vi "Vision Processing.vi"(4 "error in (no error)":errorcluster, 7 "Image Size":T1=enum."320x240") -> ()   [LabVIEW 2015]
doc: "This VI runs in parallel to other tasks. It gets images from the camera, processes them for color or shape and use that information to affect robot behavior."
uses:
  Support Vision Code/Camera Types.ctl
  <vilib>/Rock Robotics/WPI/Camera/WPI_CameraImageSize.ctl
  <userlib>/836-Library/System/QCP Support Code/QCP_Get_DBL.vi
  <userlib>/836-Library/System/QCP Support Code/QCP_Get_STR.vi
  <vilib>/Rock Robotics/Network Tables/NT Read Boolean.vi
  <userlib>/836-Library/System/QCP Support Code/QCP_Set_DBL.vi
  <vilib>/Rock Robotics/Network Tables/NT Write String.vi
  <vilib>/Rock Robotics/Network Tables/NT Write Number.vi
  <vilib>/Rock Robotics/Network Tables/NT Read Number.vi
  <vilib>/Rock Robotics/Network Tables/NT Read String.vi
  <vilib>/Rock Robotics/Network Tables/NT Write Boolean.vi
  Robot Global Data.vi
  <vilib>/vision/NI_Vision_Development_Module.lvlib
panel:
  out "Right Target":dbl
  out "Left Target":dbl
  out "Target Angle":dbl
  in  "Sideways Camera":bool
  in  "Boresight":dbl format="%#_13g"
  out "Found Targets":T2(array[cluster])=[{"Bounding box"={"left"=112.0, "top"=150.0, "right"=139.0, "bottom"=174.0}, "Aspect Ratio"=70.3125, "Area to CH"=96.83972911963883, "X Mask"=77.77777777777779, "Y Mask"=70.83333333333334, "Moment"=69.2156660279794}]
  out "FPS":dbl=5.212996497577636
  out "Qualified Particles":i32=2
  in  "Score Threshold":dbl=70.0
  in  "Aspect Fudge Factor":dbl=1.0
  in  "Min Score Threshold":dbl=75.0
  in  "Camera Type":T3=enum."MS HD3000 square"
  in  "Emphasize Limit Tests":bool
  out "Masked":T4(plugin-control)
  out "Original Image":T4(plugin-control)
  in  "Display Original":bool=TRUE
  out "Sorted Particle Scores":T5(array[cluster])=[{"Rectangle px"={"Numeric"=112.0, "Numeric 2"=150.0, "Numeric 3"=139.0, "Numeric 5"=174.0}, "Aspect Ratio"=70.3125, "Area to CH"=96.83972911963883, "X"=77.77777777777779, "Y"=70.83333333333334, "Moment Factor"=69.2156660279794}] {"Moment Factor" format="%#_3g"; "Aspect Ratio" format="%#_3g"; "Area to CH" format="%#_3g"; "X" format="%#_3g"; "Y" format="%#_3g"}
  out "Detected Targets":T6(array[cluster])=[{"Distance (ft)"=26.324888830153935, "Center"={-0.3966346153846153, -0.35}, "Normalized Rect"={"Numeric"=-0.46153846153846145, "Numeric 2"=-0.25, "Numeric 3"=-0.33173076923076916, "Numeric 5"=-0.44999999999999996}}] {"Normalized Rect"."Numeric 5" format="%#_2g"; "Normalized Rect"."Numeric 3" format="%#_2g"; "Normalized Rect"."Numeric 2" format="%#_2g"; "Normalized Rect"."Numeric" format="%#_2g"}
  in  "LED Color":T7={"Hue"={152.2312396148097, 250.0}, "Sat"={154.82142857142858, 255.0}, "Val"={100.17857142857143, 255.0}} {"Hue" scale=0.0..255.0 scale format="%#_3g"}
  # "Density Profile"
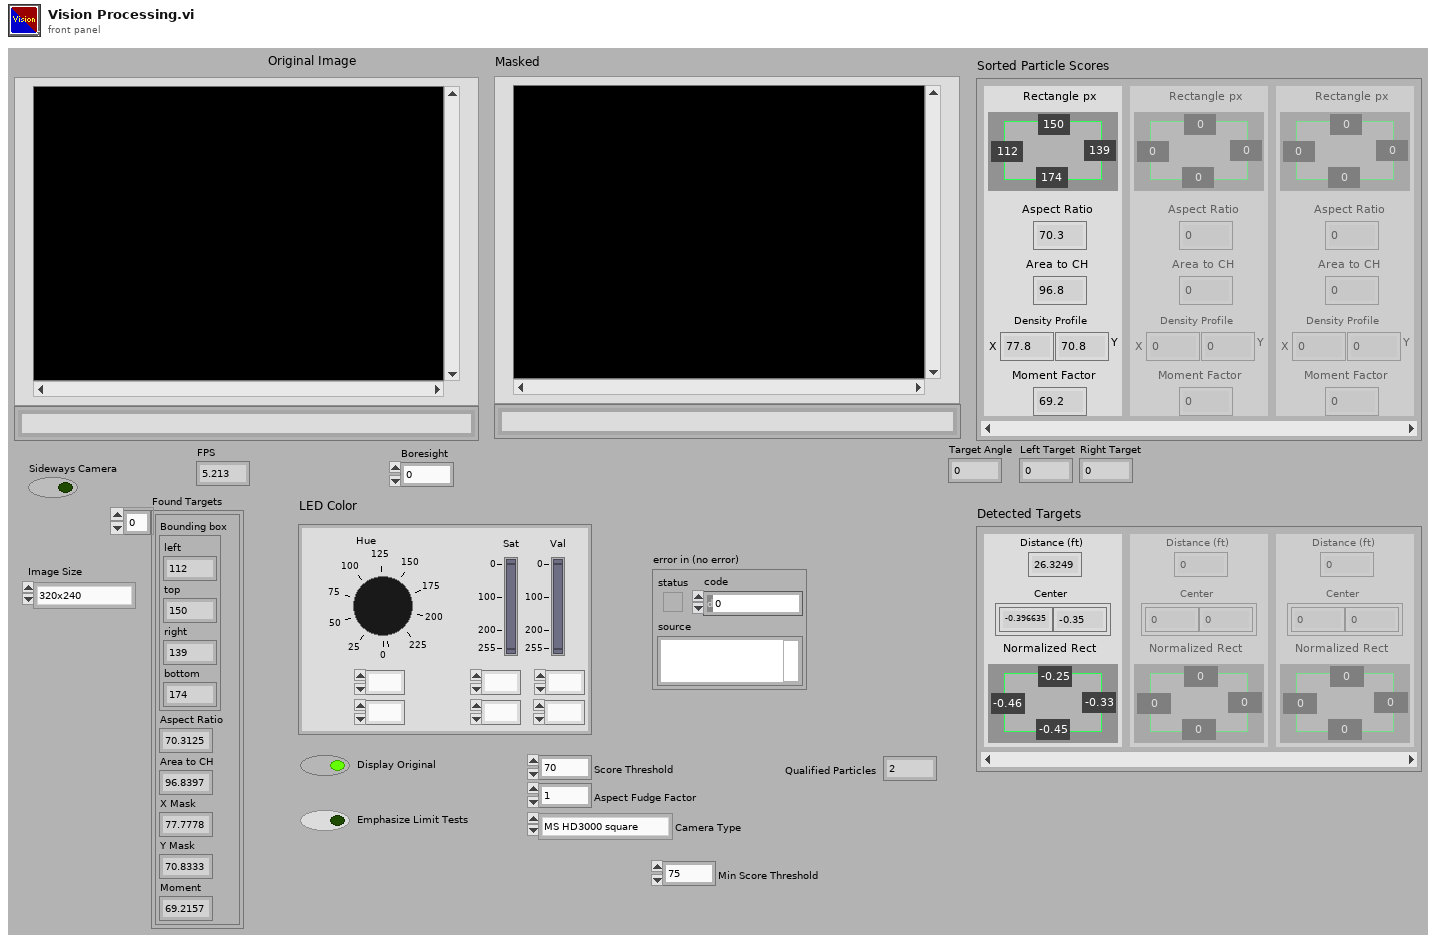
[diagram p1: front panel]
types:
  T1 = typedef "WPI_CameraImageSize.ctl" = enum16{"640x480", "320x240", "160x120", "Custom"}
  T2 = cluster{"Bounding box":cluster{"left":dbl, "top":dbl, "right":dbl, "bottom":dbl}, "Aspect Ratio":dbl, "Area to CH":dbl, "X Mask":dbl, "Y Mask":dbl, "Moment":dbl}[]
  T3 = typedef "Camera Types.ctl" = enum16{"206", "1011", "1013", "MS HD3000 square", "MS HD3000 640x480"}
  T4 = typedef "IMAQ Image.ctl" = refnum<image>
  T5 = cluster{"Rectangle px":cluster{"Numeric":dbl, "Numeric 2":dbl, "Numeric 3":dbl, "Numeric 5":dbl}, "Aspect Ratio":dbl, "Area to CH":dbl, "X":dbl, "Y":dbl, "Moment Factor":dbl}[]
  T6 = cluster{"Distance (ft)":dbl, "Center":cluster{dbl, dbl}, "Normalized Rect":cluster{"Numeric":dbl, "Numeric 2":dbl, "Numeric 3":dbl, "Numeric 5":dbl}}[]
  T7 = cluster{"Hue":cluster{dbl, dbl}, "Sat":cluster{dbl, dbl}, "Val":cluster{dbl, dbl}}
  T8 = typedef "Particle Parameters" = i32
  T9 = typedef "Image Type" = u32
  T10 = typedef "QCP Data Block.ctl" = refnum<data-value>
  T11 = typedef "WPI_CameraDevRef.ctl" = cluster{"Camera Address":string, "CameraStatus":errorcluster}
  T12 = typedef "TDMS Channel Info.ctl" = cluster{"TDMS Data":T13, "TDMS RT FIFO":refnum<k33>}
  T13 = typedef "TDMS RT FIFO Packet.ctl" = cluster{"Group/CMD":i32, "Data":dbl, "Channel":i32}
  T14 = cluster{cluster{"Value Out":dbl, "Value Out":dbl}, cluster{"Value Out":dbl, "Value Out":dbl}, cluster{"Value Out":dbl, "Value Out":dbl}}
  T15 = typedef "Drive Code Bundle.ctl" = cluster{"Sensor Data":T16, "Drive Command rt fifo":refnum<k33>}
  T16 = typedef "Sensor Cluster.ctl" = cluster{"Gyro Data":cluster{"Gyro RT FIFO":refnum<k33>, "Gyro Current":dbl, "Gyro Hold":dbl}, "Encoder Data":cluster{"Encoder RT FIFO":refnum<k33>, "Encoder Current":dbl, "Encoder Hold":dbl}, "Camera Data":cluster{"Camera RT FIFO":refnum<k33>, "Camera Current":T17}}
  T17 = typedef "Camera Cluster.ctl" = cluster{" Angle":dbl, "Valid":bool}
  T18 = cluster{"Rectangle":cluster{"Numeric":dbl, "Numeric 2":dbl, "Numeric 3":dbl, "Numeric 5":dbl}, "L":dbl, "Area to CH":dbl, "X":dbl, "Y":dbl, "Moment Factor":dbl}[]
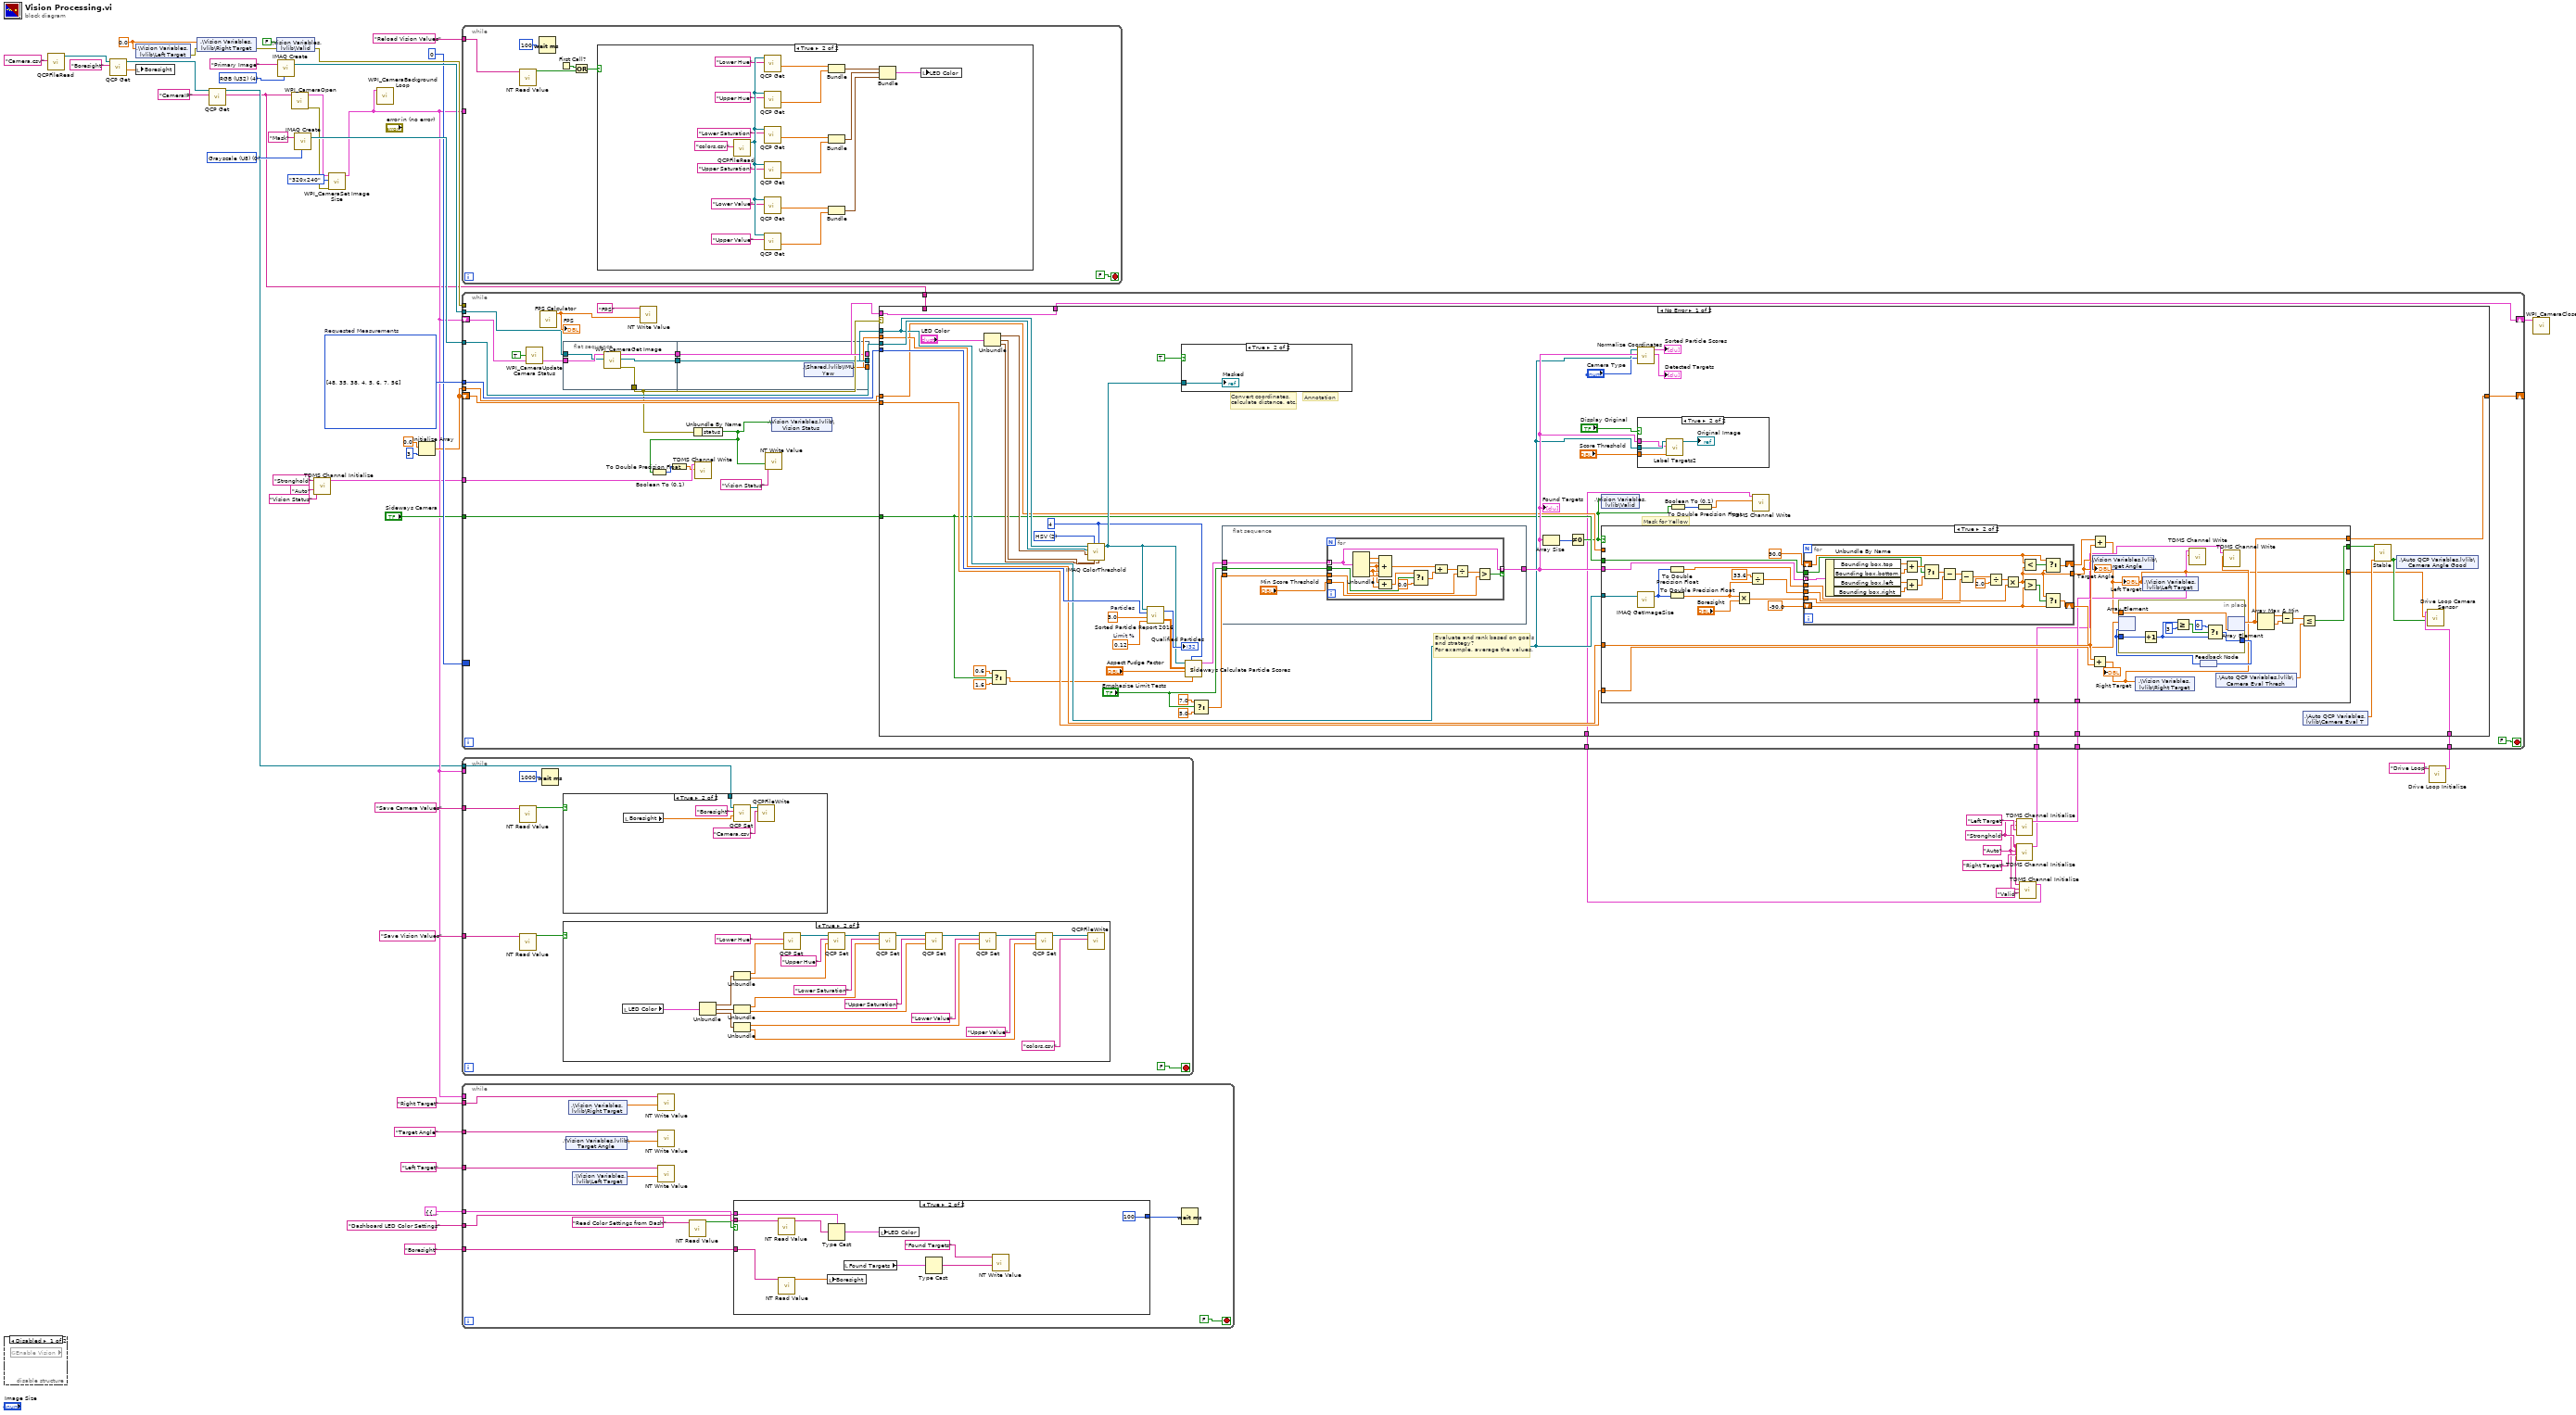
[diagram p0: block diagram]
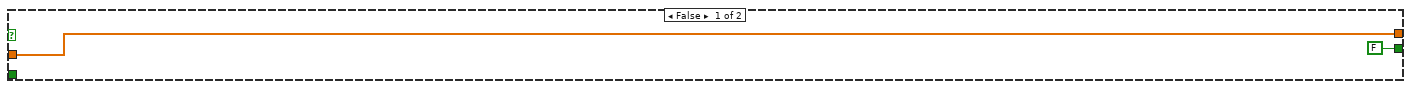
[diagram p5: hidden frame]
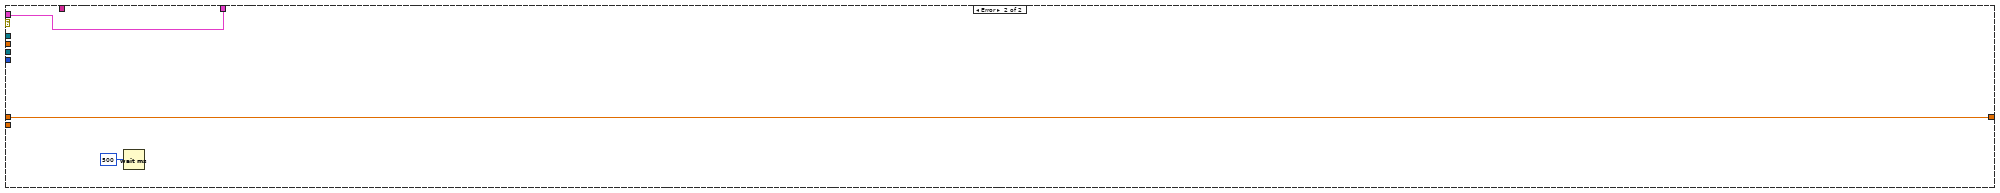
[diagram p6: hidden frame]
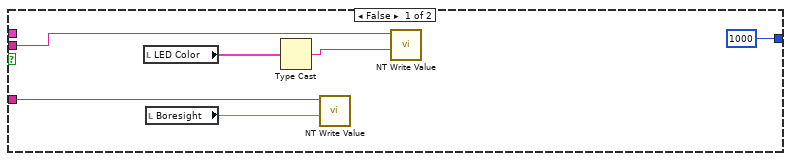
[diagram p7: hidden frame]
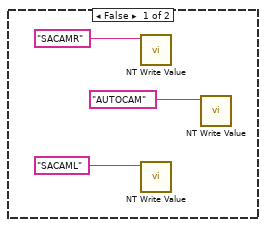
[diagram p8: hidden frame]
diagram:
  w7 = "Auto" ("Group")
  w8 = "Stronghold" ("TDMS Name")
  w30 = T8[] [48, 35, 38, 4, 5, 6, 7, 56] items=["Center of Mass X", "Center of Mass Y", "First Pixel X", "First Pixel Y", "Bounding Rect Left", "Bounding Rect Top", "Bounding Rect Right", "Bounding Rect Bottom", "Max Feret Diameter Start X", "Max Feret Diameter Start Y", "Max Feret Diameter End X", "Max Feret Diameter End Y", "Max Horiz. Segment Length Left", "Max Horiz. Segment Length Right", "Max Horiz. Segment Length Row", "-", "Bounding Rect Width", "Bounding Rect Height", "Bounding Rect Diagonal", "Perimeter", "Convex Hull Perimeter", "Holes' Perimeter", "Max Feret Diameter", "Equivalent Ellipse Major Axis", "Equivalent Ellipse Minor Axis", "Equivalent Ellipse Minor Axis (Feret)", "Equivalent Rect Long Side", "Equivalent Rect Short Side", "Equivalent Rect Diagonal", "Equivalent Rect Short Side (Feret)", "Average Horiz. Segment Length", "Average Vert. Segment Length", "Hydraulic Radius", "Waddel Disk Diameter", "-", "Area", "Holes' Area", "Particle & Holes' Area", "Convex Hull Area", "Image Area", "-", "Number of Holes", "Number of Horiz. Segments", "Number of Vert. Segments", "-", "Orientation", "Max Feret Diameter Orientation", "-", "% Area/Image Area", "% Area/(Particle & Holes' Area)", "Ratio of Equivalent Ellipse Axes", "Ratio of Equivalent Rect Sides", "-", "Elongation Factor", "Compactness Factor", "Heywood Circularity Factor", "Type Factor", "-", "Sum X", "Sum Y", "Sum XX", "Sum XY", "Sum YY", "Sum XXX", "Sum XXY", "Sum XYY", "Sum YYY", "-", "Moment of Inertia XX", "Moment of Inertia XY", "Moment of Inertia YY", "Moment of Inertia XXX", "Moment of Inertia XXY", "Moment of Inertia XYY", "Moment of Inertia YYY", "Norm. Moment of Inertia XX", "Norm. Moment of Inertia XY", "Norm. Moment of Inertia YY", "Norm. Moment of Inertia XXX", "Norm. Moment of Inertia XXY", "Norm. Moment of Inertia XYY", "Norm. Moment of Inertia YYY", "Hu Moment 1", "Hu Moment 2", "Hu Moment 3", "Hu Moment 4", "Hu Moment 5", "Hu Moment 6", "Hu Moment 7"]  # Requested Measurements
  w41 = 0.0 ("Left Target")
  w49 = T9 0 items=["Grayscale (U8)", "Grayscale (I16)", "Grayscale (SGL)", "Complex (CSG)", "RGB (U32)", "HSL (U32)", "RGB (U64)", "Grayscale (U16)"] ("Image Type")
  w52 = T9 4 items=["Grayscale (U8)", "Grayscale (I16)", "Grayscale (SGL)", "Complex (CSG)", "RGB (U32)", "HSL (U32)", "RGB (U64)"] ("Image Type")
  n1 = disable-structure shown="Disabled" {
    frame Disabled {
      n2 = global read "Robot Global Data.vi" "Enable Vision"() -> ()  [unwired: 1 out]
    }
    frame Enabled {
    }
  }
  n3 = call <userlib>:"QCPFileRead.vi"("File Path"="Camera.csv") -> ("QCP Data Block Out"=w29:T10)  [unwired: 9 in, 1 out]
  n4 = call-poly <userlib>:"QCP Get.vi"("QCP Data Block In"=w29, "QCP Name"="Boresight") -> ("QCP Data Block Out"=w22:T10, "Value Out"=w35:dbl)  [unwired: 6 in, 1 out]
  n5 = shared-variable ".\\Vision Variables.lvlib\\Left Target"(w41) -> (error out=w32:errorcluster)  [unwired: 1 in]
  n6 = local write "Boresight"(w35) -> ()
  n7 = shared-variable ".\\Vision Variables.lvlib\\Right Target"(w41, error in=w32) -> (error out=w31:errorcluster)
  n8 = call-poly <userlib>:"QCP Get.vi"("QCP Data Block In"=w22, "QCP Name"="CameraIP") -> ("QCP Data Block Out"=w16:T10, "Value Out"=w15:string)  [unwired: 6 in, 1 out]
  n9 = shared-variable ".\\Vision Variables.lvlib\\Valid"(FALSE ("Valid"), error in=w31) -> (error out=w33:errorcluster)
  n10 = call "IMAQ Create"("Image Name"="Primary Image", "Image Type"=w52) -> ("New Image"=w50:T4)  [unwired: 2 in, 2 out]
  n11 = call <vilib>:"WPI_CameraOpen.vi"("Camera Address"=w15) -> ("error out"=w18:errorcluster, "CameraDevRef"=w20:T11)  [unwired: 9 in]
  n12 = call "IMAQ Create"("Image Name"="Mask", "Image Type"=w49) -> ("New Image"=w47:T4)  [unwired: 2 in, 2 out]
  n13 = call <userlib>:"TDMS Channel Initialize.vi"("Channel"="Vision Status", "Group"="Auto", "TDMS"="Stronghold") -> ("TDMS Channel Info"=w1:T12)  [unwired: 8 in]
  n14 = call <vilib>:"WPI_CameraSet Image Size.vi"("error in (no error)"=w18, "Image Size"=WPI_CameraImageSize."320x240", "CameraDevRef"=w20) -> ("CameraDevRef Out"=w19:T11)  [unwired: 7 in, 1 out]
  n15 = call <vilib>:"WPI_CameraBackground Loop.vi"("CameraDevRef"=w19) -> ()  [unwired: 11 in]
  n16 = Initialize Array(0.0, 3 ("dimension size")) -> (w24:dbl[])
  n17 = while {
    tunnel: w19 -> [_]
    tunnel: "Reload Vision Values" ("Name") -> [w54]
    stop <- FALSE stop-if-true
    n18 = call-poly <vilib>:"NT Read Value.vi"("Name"=w54) -> ("Boolean"=w56:bool)  [unwired: 9 in, 1 out]
    n19 = Wait (ms)(milliseconds to wait=u32 100) -> ()  [unwired: 1 out]
    n20 = First Call?() -> (First Call?: T/F=w57:bool)
    n21 = Or(x=w57, y=w56) -> (x .or. y?=w55:bool)
    n22 = case shown="True" w55 {
      frame False {
      }
      frame True {
        n23 = call <userlib>:"QCPFileRead.vi"("File Path"="colors.csv") -> ("QCP Data Block Out"=w77:T10)  [unwired: 9 in, 1 out]
        n24 = call-poly <userlib>:"QCP Get.vi"("QCP Data Block In"=w77, "QCP Name"="Lower Hue") -> ("Value Out"=w69:dbl)  [unwired: 6 in, 2 out]
        n25 = call-poly <userlib>:"QCP Get.vi"("QCP Data Block In"=w77, "QCP Name"="Upper Hue") -> ("Value Out"=w68:dbl)  [unwired: 6 in, 2 out]
        n26 = call-poly <userlib>:"QCP Get.vi"("QCP Data Block In"=w77, "QCP Name"="Lower Saturation") -> ("Value Out"=w66:dbl)  [unwired: 6 in, 2 out]
        n27 = call-poly <userlib>:"QCP Get.vi"("QCP Data Block In"=w77, "QCP Name"="Upper Saturation") -> ("Value Out"=w65:dbl)  [unwired: 6 in, 2 out]
        n28 = call-poly <userlib>:"QCP Get.vi"("QCP Data Block In"=w77, "QCP Name"="Lower Value") -> ("Value Out"=w62:dbl)  [unwired: 6 in, 2 out]
        n29 = call-poly <userlib>:"QCP Get.vi"("QCP Data Block In"=w77, "QCP Name"="Upper Value") -> ("Value Out"=w61:dbl)  [unwired: 6 in, 2 out]
        n30 = Bundle("Value Out"=w69, "Value Out"=w68) -> (w67:cluster{"Value Out":dbl, "Value Out":dbl})  [unwired: 1 in]
        n31 = Bundle("Value Out"=w66, "Value Out"=w65) -> (w64:cluster{"Value Out":dbl, "Value Out":dbl})  [unwired: 1 in]
        n32 = Bundle("Value Out"=w62, "Value Out"=w61) -> (w63:cluster{"Value Out":dbl, "Value Out":dbl})  [unwired: 1 in]
        n33 = Bundle(w67, w64, w63) -> (w60:T14)  [unwired: 1 in]
        n34 = local write "LED Color"(w60) -> ()
      }
    }
  }
  n35 = while {
    tunnel: w19 -> [_]
    tunnel: "Save Camera Values" ("Name") -> [w80]
    tunnel: "Save Vision Values" ("Name") -> [w79]
    tunnel: w16 -> [w78]
    stop <- FALSE stop-if-true
    n36 = call-poly <vilib>:"NT Read Value.vi"("Name"=w80) -> ("Boolean"=w81:bool)  [unwired: 9 in, 1 out]
    n37 = call-poly <vilib>:"NT Read Value.vi"("Name"=w79) -> ("Boolean"=w82:bool)  [unwired: 9 in, 1 out]
    n38 = Wait (ms)(milliseconds to wait=u32 1000) -> ()  [unwired: 1 out]
    n39 = case shown="True" w81 {
      tunnel: w78 -> [_ w88]
      frame False {
        n40 = call-poly <vilib>:"NT Write Value.vi"("Name"="SACAMR") -> ()  [unwired: 10 in, 1 out]
        n41 = call-poly <vilib>:"NT Write Value.vi"("Name"="SACAML") -> ()  [unwired: 10 in, 1 out]
        n42 = call-poly <vilib>:"NT Write Value.vi"("Name"="AUTOCAM") -> ()  [unwired: 10 in, 1 out]
      }
      frame True {
        n43 = local read "Boresight"() -> (w90:dbl)
        n44 = call-poly <userlib>:"QCP Set.vi"("QCP Data Block In"=w88, "QCP Name"="Boresight", "Value In"=w90) -> ("QCP Data Block Out"=w89:T10)  [unwired: 7 in]
        n45 = call <userlib>:"QCPFileWrite.vi"("File Path"="Camera.csv", "QCP Data Block In"=w89) -> ()  [unwired: 8 in, 2 out]
      }
    }
    n46 = case shown="True" w82 {
      frame False {
      }
      frame True {
        n47 = local read "LED Color"() -> (w102:T7)
        n48 = Unbundle(w102) -> ("Hue"=w101:cluster{dbl, dbl}, "Sat"=w100:cluster{dbl, dbl}, "Val"=w99:cluster{dbl, dbl})
        n49 = Unbundle(w101) -> (w94:dbl, w93:dbl)
        n50 = Unbundle(w100) -> (w96:dbl, w95:dbl)
        n51 = Unbundle(w99) -> (w98:dbl, w97:dbl)
        n52 = call-poly <userlib>:"QCP Set.vi"("QCP Name"="Lower Hue", "Value In"=w94) -> ("QCP Data Block Out"=w107:T10)  [unwired: 8 in]
        n53 = call-poly <userlib>:"QCP Set.vi"("QCP Data Block In"=w107, "QCP Name"="Upper Hue", "Value In"=w93) -> ("QCP Data Block Out"=w108:T10)  [unwired: 7 in]
        n54 = call-poly <userlib>:"QCP Set.vi"("QCP Data Block In"=w108, "QCP Name"="Lower Saturation", "Value In"=w96) -> ("QCP Data Block Out"=w106:T10)  [unwired: 7 in]
        n55 = call-poly <userlib>:"QCP Set.vi"("QCP Data Block In"=w106, "QCP Name"="Upper Saturation", "Value In"=w95) -> ("QCP Data Block Out"=w105:T10)  [unwired: 7 in]
        n56 = call-poly <userlib>:"QCP Set.vi"("QCP Data Block In"=w105, "QCP Name"="Lower Value", "Value In"=w98) -> ("QCP Data Block Out"=w104:T10)  [unwired: 7 in]
        n57 = call-poly <userlib>:"QCP Set.vi"("QCP Data Block In"=w104, "QCP Name"="Upper Value", "Value In"=w97) -> ("QCP Data Block Out"=w103:T10)  [unwired: 7 in]
        n58 = call <userlib>:"QCPFileWrite.vi"("File Path"="colors.csv", "QCP Data Block In"=w103) -> ()  [unwired: 8 in, 2 out]
      }
    }
  }
  n59 = while {
    tunnel: "Dashboard LED Color Settings" ("Name") -> [w125]
    tunnel: T7 {"Hue"={152.2312396148097, 250.0}, "Sat"={154.82142857142858, 255.0}, "Val"={100.17857142857143, 255.0}} ("LED Color") -> [w124]
    tunnel: w19 -> [_]
    tunnel: "Left Target" ("Name") -> [w120]
    tunnel: "Right Target" ("Name") -> [w119]
    tunnel: "Boresight" ("Name") -> [w118]
    tunnel: "Target Angle" ("Name") -> [w116]
    stop <- FALSE stop-if-true
    n60 = shared-variable ".\\Vision Variables.lvlib\\Target Angle"() -> (w117:dbl)  [unwired: 1 in, 1 out]
    n61 = shared-variable ".\\Vision Variables.lvlib\\Right Target"() -> (w121:dbl)  [unwired: 1 in, 1 out]
    n62 = shared-variable ".\\Vision Variables.lvlib\\Left Target"() -> (w122:dbl)  [unwired: 1 in, 1 out]
    n63 = call-poly <vilib>:"NT Write Value.vi"("Numeric"=w121, "Name"=w119) -> ()  [unwired: 9 in, 1 out]
    n64 = call-poly <vilib>:"NT Write Value.vi"("Numeric"=w117, "Name"=w116) -> ()  [unwired: 9 in, 1 out]
    n65 = call-poly <vilib>:"NT Write Value.vi"("Numeric"=w122, "Name"=w120) -> ()  [unwired: 9 in, 1 out]
    n66 = call-poly <vilib>:"NT Read Value.vi"("Name"="Read Color Settings from Dash") -> ("Boolean"=w126:bool)  [unwired: 9 in, 1 out]
    n67 = case shown="True" w126 {
      tunnel: w125 -> [w133 w142]
      tunnel: w124 -> [_ w141]
      tunnel: [u32 1000 ("milliseconds to wait") u32 100 ("milliseconds to wait")] -> w123
      tunnel: w118 -> [w130 w136]
      frame False {
        n68 = local read "LED Color"() -> (w134:T7)
        n69 = local read "Boresight"() -> (w129:dbl)
        n70 = Type Cast(x=w134) -> (*(type *) &x=w132:string)  [unwired: 1 in]
        n71 = call-poly <vilib>:"NT Write Value.vi"("Numeric"=w129, "Name"=w130) -> ()  [unwired: 9 in, 1 out]
        n72 = call-poly <vilib>:"NT Write Value.vi"("String"=w132, "Name"=w133) -> ()  [unwired: 9 in, 1 out]
      }
      frame True {
        n73 = call-poly <vilib>:"NT Read Value.vi"("Name"=w142) -> ("String"=w143:string)  [unwired: 9 in, 1 out]
        n74 = call-poly <vilib>:"NT Read Value.vi"("Name"=w136) -> ("Numeric"=w135:dbl)  [unwired: 9 in, 1 out]
        n75 = local write "Boresight"(w135) -> ()
        n76 = Type Cast(type=w141, x=w143) -> (*(type *) &x=w144:T7)
        n77 = local read "Found Targets"() -> (w140:T2)
        n78 = local write "LED Color"(w144) -> ()
        n79 = Type Cast(x=w140) -> (*(type *) &x=w139:string)  [unwired: 1 in]
        n80 = call-poly <vilib>:"NT Write Value.vi"("String"=w139, "Name"="Found Targets") -> ()  [unwired: 9 in, 1 out]
      }
    }
    n81 = Wait (ms)(milliseconds to wait=w123) -> ()  [unwired: 1 out]
  }
  n82 = call <userlib>:"TDMS Channel Initialize.vi"("Channel"="Left Target", "Group"=w7, "TDMS"=w8) -> ("TDMS Channel Info"=w10:T12)  [unwired: 8 in]
  n83 = call <userlib>:"TDMS Channel Initialize.vi"("Channel"="Right Target", "Group"=w7, "TDMS"=w8) -> ("TDMS Channel Info"=w9:T12)  [unwired: 8 in]
  n84 = call <userlib>:"TDMS Channel Initialize.vi"("Channel"="Valid", "Group"=w7, "TDMS"=w8) -> ("TDMS Channel Info"=w5:T12)  [unwired: 8 in]
  n85 = call <userlib>:"Drive Loop Initialize.vi"("name (unnamed)"="Drive Loop") -> ("Drive Loop Cluster"=w14:T15)  [unwired: 9 in, 1 out]
  n86 = while {
    shift-right: [w157] -> w46
    shift-left: w19 -> [w159]
    tunnel: w50 -> [w171]
    tunnel: w47 -> [w164]
    tunnel: w30 -> [w170]
    tunnel: w33 -> [_]
    border: 0 -> [_]
    shift-right: [w163] -> _
    shift-left: w24 -> [w162]
    tunnel: w24 -> [w161]
    tunnel: "Sideways Camera" -> [w160]
    tunnel: w15 -> [w156]
    tunnel: w14 -> [w152]
    tunnel: w10 -> [w151]
    tunnel: w9 -> [w150]
    tunnel: w5 -> [w149]
    tunnel: w1 -> [w148]
    stop <- FALSE stop-if-true
    n87 = call <vilib>:"WPI_CameraUpdate Camera Status.vi"("CameraDevRef In"=w159, "Enable Vision"=TRUE) -> ("CameraDevRef Out"=w169:T11)  [unwired: 3 in]
    n88 = call <userlib>:"FPS Calculator.vi"() -> ("FPS"=w173:dbl)  [unwired: 11 in]
    "FPS" <- w173
    n89 = flat-sequence {
      tunnel: w169 -> [w317]
      tunnel: w171 -> [w316]
      tunnel: [w315] -> w168
      tunnel: [w314] -> w167
      tunnel: [w313] -> w155
      tunnel: [w319] -> w166
      tunnel: [w320] -> w158
      tunnel: w168 -> [w320]
      tunnel: w167 -> [w319]
      tunnel: [w318] -> w165
      frame #0 {
        n90 = call <vilib>:"WPI_CameraGet Image.vi"("Image"=w316, "CameraDevRef"=w317) -> ("error out"=w313:errorcluster, "Image Out"=w314:T4, "CameraDevRef Out"=w315:T11)  [unwired: 7 in]
      }
      frame #1 {
        n91 = shared-variable ".\\Shared.lvlib\\IMU Yaw"() -> (w318:dbl)  [unwired: 1 in, 1 out]
      }
    }
    n92 = call-poly <vilib>:"NT Write Value.vi"("Numeric"=w173, "Name"="FPS") -> ()  [unwired: 9 in, 1 out]
    n93 = Unbundle By Name(w155) -> ("status"=w147:bool)
    n94 = Boolean To (0,1)(Boolean=w147) -> (0, 1=w146:i16)
    n95 = To Double Precision Float(number=w146) -> (double precision float=w145:dbl)
    n96 = call <userlib>:"TDMS Channel Write.vi"("Data"=w145, "TDMS Channel Info in"=w148) -> ()  [unwired: 10 in]
    n97 = call-poly <vilib>:"NT Write Value.vi"("Boolean"=w147, "Name"="Vision Status") -> ()  [unwired: 9 in, 1 out]
    n98 = shared-variable ".\\Vision Variables.lvlib\\Vision Status"(w147) -> ()  [unwired: 1 in, 1 out]
    n99 = case shown="No Error" w155 {
      tunnel: w164 -> [w222 _]
      tunnel: w170 -> [w218 _]
      tunnel: w166 -> [w202 _]
      tunnel: w165 -> [w201 _]
      tunnel: w162 -> [w198 _]
      tunnel: [w196 w312] -> w163
      tunnel: w161 -> [w195 w312]
      tunnel: w160 -> [w191 _]
      tunnel: w158 -> [w184 w311]
      tunnel: [w184 w311] -> w157
      tunnel: w156 -> [_ _]
      tunnel: w152 -> [w183 _]
      tunnel: w151 -> [w180 _]
      tunnel: w150 -> [w179 _]
      tunnel: w149 -> [w175 _]
      frame No Error {
        w206 = 4 ("Replace Value")
        w214 = u16 2 items=["RGB", "HSL", "HSV", "HSI"] ("Color Mode")
        w215 = 0.12  # Limit %
        w217 = 3.0  # Particles
        # "Convert coordinates,\ncalculate distance, etc."
        # "Annotation"
        # "Evaluate and rank based on goals\nand strategy?\nFor example, average the values."
        # "Mask for Yellow"
        n100 = Unbundle("LED Color") -> ("Hue"=w221:cluster{dbl, dbl}, "Sat"=w220:cluster{dbl, dbl}, "Val"=w219:cluster{dbl, dbl})
        n101 = Select(t=0.6 ("Expected Aspect Ratio"), s=w191, f=1.6) -> (s? t:f=w193:dbl)
        n102 = call "IMAQ ColorThreshold"("Blue or Luma or Val or Inten Range"=w219, "Replace Value"=w206, "Green or Sat Range"=w220, "Color Mode"=w214, "Red or Hue Range"=w221, "Image Dst"=w222, "Image Src"=w202) -> ("Image Dst Out"=w213:T4)  [unwired: 3 in, 1 out]
        n103 = call "Sorted Particle Report 2016.vi"("Min Area Size %"=w215, "Particle Count Limit"=w217, "Pixel Measurements"=w218, "Image in"=w213) -> ("Sorted Data"=w212:dbl[][], "Particles"=→"Qualified Particles":i32)
        n104 = case shown="True" TRUE ("Display Mask") {
          tunnel: w213 -> [_ w227]
          frame False {
          }
          frame True {
            "Masked" <- w227
          }
        }
        n105 = call "Sideways Calculate Particle Scores.vi"("Expected Aspect Ratio"=w193, "Pixel Value"=w206, "Aspect Fudge Factor"="Aspect Fudge Factor", "Sorted Data"=w212, "Image in"=w213) -> ("Scores"=w210:T2)  [unwired: 6 in]
        n106 = Select(t=7.0, s="Emphasize Limit Tests", f=5.0) -> (s? t:f=w207:dbl)
        n107 = flat-sequence {
          tunnel: w210 -> [w232]
          tunnel: w207 -> [w230]
          tunnel: [w228] -> w204
          tunnel: "Emphasize Limit Tests" -> [w231]
          frame #0 {
            n108 = for {
              tunnel: w232 -> [w246] mode=indexing
              tunnel: [w246] -> w228 mode=indexing if=w245
              tunnel: w230 -> [w243]
              tunnel: "Min Score Threshold" -> [w242]
              tunnel: w231 -> [w235]
              n109 = Unbundle(w246) -> ("Aspect Ratio"=w248:dbl, "Area to CH"=w247:dbl, "X Mask"=w237:dbl, "Y Mask"=w238:dbl, "Moment"=w239:dbl)  [unwired: 1 out]
              n110 = Compound Arithmetic op=ADD(w248, w247, w237, w238, w239) -> (w241:dbl)
              n111 = Compound Arithmetic op=ADD(w237, w238) -> (w236:dbl)
              n112 = Select(t=w236, s=w235, f=0.0) -> (s? t:f=w234:dbl)
              n113 = Compound Arithmetic op=ADD(w241, w234) -> (w240:dbl)
              n114 = Divide(x=w240, y=w243) -> (x/y=w244:dbl)
              n115 = Greater?(x=w244, y=w242) -> (0:w245:bool)
            }
          }
        }
        n116 = Array Size(array=w204) -> (size(s)=w203:i32)
        n117 = Not Equal To 0?(x=w203) -> (x != 0?=w177:bool)
        n118 = shared-variable ".\\Vision Variables.lvlib\\Valid"(w177) -> ()  [unwired: 1 in, 1 out]
        n119 = case shown="True" w177 {
          tunnel: w204 -> [_ w279]
          tunnel: w201 -> [_ w278]
          tunnel: w202 -> [_ w271]
          tunnel: w198 -> [_ w264]
          tunnel: [FALSE w257] -> w197
          tunnel: [w249 w256] -> w196
          tunnel: w195 -> [w249 _]
          tunnel: w191 -> [_ w255]
          tunnel: [_ w251] -> w181
          tunnel: w180 -> [_ w254]
          tunnel: w179 -> [_ w253]
          frame False {
          }
          frame True {
            n120 = call "IMAQ GetImageSize"("Image"=w271) -> ("Y Resolution"=w269:i32)  [unwired: 3 in, 2 out]
            n121 = To Double Precision Float(number=w269) -> (double precision float=w270:dbl)
            n122 = To Double Precision Float(number=w269) -> (double precision float=w267:dbl)
            n123 = Multiply(x=w267, y="Boresight") -> (x*y=w266:dbl)
            n124 = Divide(x=33.6, y=w267) -> (x/y=w272:dbl)
            n125 = for {
              tunnel: w279 -> [w309] mode=indexing
              tunnel: w270 -> [w306]
              tunnel: w272 -> [w305]
              shift-right: [w302] -> w274
              shift-left: -90.0 -> [w300]
              shift-right: [w301] -> w275
              shift-left: 90.0 -> [w297]
              tunnel: w266 -> [w295]
              tunnel: [w293] -> w265
              tunnel: w255 -> [w288]
              n126 = Unbundle By Name(w309) -> ("Bounding box.top"=w308:dbl, "Bounding box.bottom"=w307:dbl, "Bounding box.left"=w291:dbl, "Bounding box.right"=w292:dbl)
              n127 = Add(x=w308, y=w307) -> (x+y=w290:dbl)
              n128 = Add(x=w291, y=w292) -> (x+y=w289:dbl)
              n129 = Select(t=w290, s=w288, f=w289) -> (s? t:f=w287:dbl)
              n130 = Subtract(x=w287, y=w306) -> (x-y=w296:dbl)
              n131 = Subtract(x=w296, y=w295) -> (x-y=w294:dbl)
              n132 = Divide(x=w294, y=2.0) -> (x/y=w298:dbl)
              n133 = Multiply(x=w298, y=w305) -> (x*y=w293:dbl)
              n134 = Less?(x=w297, y=w293) -> (x < y?=w304:bool)
              n135 = Greater?(x=w293, y=w300) -> (0:w303:bool)
              n136 = Select(t=w297, s=w304, f=w293) -> (s? t:f=w301:dbl)
              n137 = Select(t=w293, s=w303, f=w300) -> (s? t:f=w302:dbl)
            }
            "Target Angle" <- w265
            n138 = Add(x=w278, y=w274) -> (x+y=w252:dbl)
            "Right Target" <- w252
            n139 = Add(x=w275, y=w278) -> (x+y=w251:dbl)
            "Left Target" <- w251
            n140 = shared-variable ".\\Vision Variables.lvlib\\Target Angle"(w265) -> ()  [unwired: 1 in, 1 out]
            n141 = shared-variable ".\\Vision Variables.lvlib\\Right Target"(w252) -> ()  [unwired: 1 in, 1 out]
            n142 = shared-variable ".\\Vision Variables.lvlib\\Left Target"(w251) -> ()  [unwired: 1 in, 1 out]
            n143 = call <userlib>:"TDMS Channel Write.vi"("Data"=w251, "TDMS Channel Info in"=w254) -> ()  [unwired: 10 in]
            n144 = feedback #1() -> (w263:i32)
            n145 = in-place {
              in-place-border: w251 -> [w286]
              in-place-border: w263 -> [w285]
              in-place-border: [w280] -> w262
              n146 = in-place-array #2(w264, w263) -> ()  [unwired: 1 out]
              n147 = Increment(x=w285) -> (x+1=w282:i32)
              n148 = Greater Or Equal?(x=w282, y=3) -> (x >= y?=w283:bool)
              n149 = Select(t=0, s=w283, f=w282) -> (s? t:f=w280:i32)
              n150 = in-place-array #2(w286) -> (w256:dbl[])  [unwired: 1 out]
            }
            n151 = feedback-in #1(w262) -> ()
            n152 = shared-variable ".\\Auto QCP Variables.lvlib\\Camera Eval Thresh"() -> (w258:dbl)  [unwired: 1 in, 1 out]
            n153 = call <userlib>:"TDMS Channel Write.vi"("Data"=w252, "TDMS Channel Info in"=w253) -> ()  [unwired: 10 in]
            n154 = Array Max & Min(array=w256) -> (max value=w261:dbl, min value=w260:dbl)  [unwired: 2 out]
            n155 = Subtract(x=w261, y=w260) -> (x-y=w259:dbl)
            n156 = Less Or Equal?(x=w259, y=w258) -> (x <= y?=w257:bool)
          }
        }
        n157 = call "Normalize Coordinates.vi"("Camera Type"="Camera Type", "Targets"=w204, "Image in"=w202) -> ("Found Targets"=→"Detected Targets":T6, "Sorted Scores"=→"Sorted Particle Scores":T18)  [unwired: 7 in]
        n158 = case shown="True" "Display Original" {
          tunnel: w202 -> [_ w226]
          tunnel: w204 -> [_ w224]
          tunnel: "Score Threshold" -> [_ w223]
          frame False {
          }
          frame True {
            n159 = call "Label Targets2.vi"("Score Threshold"=w223, "Targets"=w224, "Image in"=w226) -> ("Image out"=→"Original Image":T4)  [unwired: 8 in]
          }
        }
        n160 = Boolean To (0,1)(Boolean=w177) -> (0, 1=w178:i16)
        n161 = To Double Precision Float(number=w178) -> (double precision float=w176:dbl)
        n162 = call <userlib>:"TDMS Channel Write.vi"("Data"=w176, "TDMS Channel Info in"=w175) -> ()  [unwired: 10 in]
        n163 = shared-variable ".\\Auto QCP Variables.lvlib\\Camera Eval T"() -> (w199:dbl)  [unwired: 1 in, 1 out]
        n164 = call <userlib>:"Stable.vi"("Eval Period (sec)"=w199, "Signal Input"=w197) -> ("Stable"=w182:bool)  [unwired: 9 in]
        n165 = shared-variable ".\\Auto QCP Variables.lvlib\\Camera Angle Good"(w182) -> ()  [unwired: 1 in, 1 out]
        n166 = call <userlib>:"Drive Loop Camera Sensor.vi"("Stable"=w182, "Numeric"=w181, "Drive Loop Cluster"=w183) -> ()  [unwired: 9 in]
        "Found Targets" <- w204
      }
      frame Error {
        n167 = Wait (ms)(milliseconds to wait=u32 500) -> ()  [unwired: 1 out]
      }
    }
  }
  n168 = call <vilib>:"WPI_CameraClose.vi"("CameraDevRef"=w46) -> ()  [unwired: 1 in, 10 out]
